vi "Generate_Feature_Layers_Name.vi"(11 "[LayerID, PatchSize]":T1) -> (3 "Layers":string)   [LabVIEW 2020]
uses:
  Controls/Feature_Layers_CFG.ctl
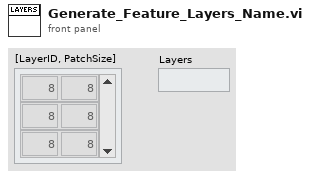
[diagram p1: front panel]
types:
  T1 = typedef "Feature_Layers_CFG.ctl" = cluster{"Layer_ID":i32, "Patch_Size":i32}[]
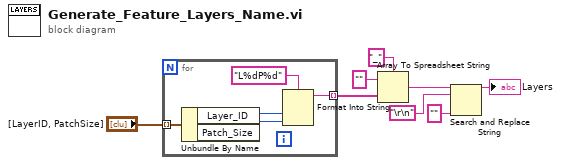
[diagram p0: block diagram]
diagram:
  n1 = for {
    tunnel: "[LayerID, PatchSize]" -> [w13] mode=indexing
    tunnel: [w9] -> w2 mode=indexing
    n2 = Unbundle By Name(w13) -> ("Layer_ID"=w12:i32, "Patch_Size"=w11:i32)
    n3 = Format Into String(format string="L%dP%d", w12, w11) -> (resulting string=w9:string)  [unwired: 2 in, 1 out]
  }
  n4 = Array To Spreadsheet String(delimiter (Tab)="_", array=w2, 3:"" ("format string")) -> (spreadsheet string=w7:string)
  n5 = Search and Replace String(input string=w7, search string="\r\n", replace string="" ("replace string (\"\")")) -> (result string=→"Layers":string)  [unwired: 5 in, 3 out]
